vi "TRI speed.vi"(9 "t2":dbl, 10 "i":i32, 11 "dt(s)":dbl) -> (0 "complet?":bool, 3 "Waveform Chart":dbl(graph))   [LabVIEW 2019]
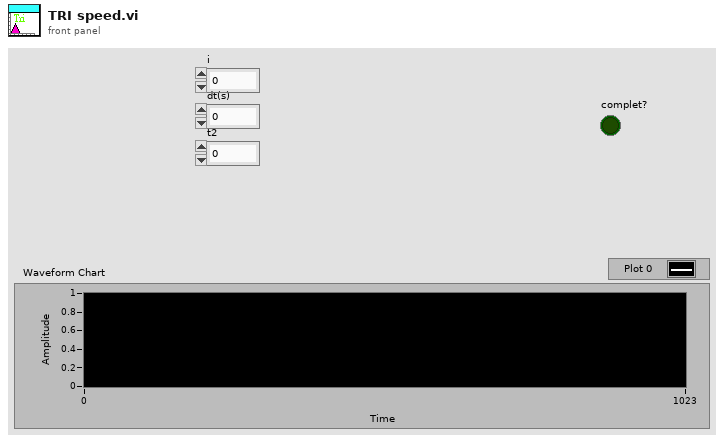
[diagram p1: front panel]
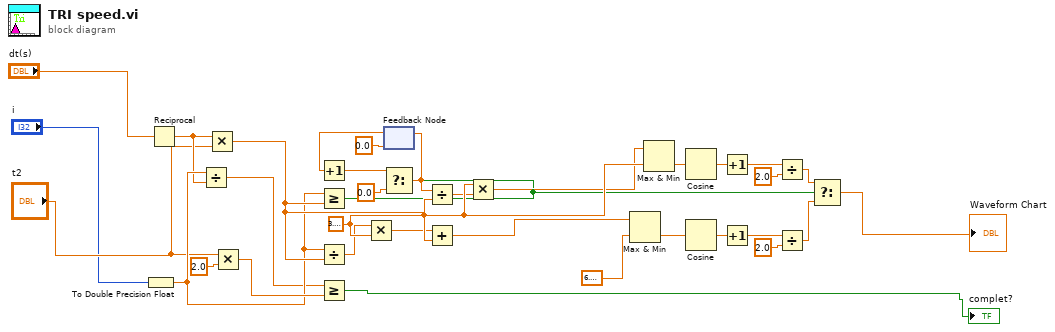
[diagram p0: block diagram]
diagram:
  w28 = 3.141592653589793
  n1 = To Double Precision Float(number="i") -> (double precision float=w9:dbl)
  n2 = Reciprocal(x="dt(s)") -> (1/x=w8:dbl)
  n3 = Divide(x=w9, y=w8) -> (x/y=w7:dbl)
  n4 = Multiply(x=w8, y="t2") -> (x*y=w13:dbl)
  n5 = Multiply(x="t2", y=2.0) -> (x*y=w11:dbl)
  n6 = Greater Or Equal?(x=w9, y=w13) -> (x >= y?=w1:bool)
  n7 = Divide(x=w9, y=w13) -> (x/y=w10:dbl)
  n8 = Greater Or Equal?(x=w7, y=w11) -> (x >= y?=→"complet?":bool)
  n9 = Multiply(x=w10, y=w28) -> (x*y=w14:dbl)
  n10 = feedback #1(0.0 ("f")) -> (w22:dbl)
  n11 = Increment(x=w22) -> (x+1=w23:dbl)
  n12 = Select(t=w23, s=w1, f=0.0) -> (s? t:f=w25:dbl)
  n13 = feedback-in #1(w25) -> ()
  n14 = Divide(x=w25, y=w13) -> (x/y=w26:dbl)
  n15 = Add(x=w14, y=w28) -> (x+y=w16:dbl)
  n16 = Multiply(x=w28, y=w26) -> (x*y=w27:dbl)
  n17 = Max & Min(x=w16, y=6.283185307179586) -> (min(x,y)=w17:dbl)  [unwired: 1 out]
  n18 = Max & Min(x=w27, y=w28) -> (min(x,y)=w29:dbl)  [unwired: 1 out]
  n19 = Cosine(x=w29) -> (cos(x)=w30:dbl)
  n20 = Cosine(x=w17) -> (cos(x)=w18:dbl)
  n21 = Increment(x=w30) -> (x+1=w31:dbl)
  n22 = Increment(x=w18) -> (x+1=w19:dbl)
  n23 = Divide(x=w31, y=2.0) -> (x/y=w34:dbl)
  n24 = Divide(x=w19, y=2.0) -> (x/y=w33:dbl)
  n25 = Select(t=w34, s=w1, f=w33) -> (s? t:f=→"Waveform Chart":dbl)
